vi "Sensor().vi"() -> (3 "Sensor.lvclass":refnum<class "Sensor.lvclass">)   [LabVIEW 2014, in "Sensors.lvlib" / "Sensor.lvclass"]
uses:
  Sensor.lvclass
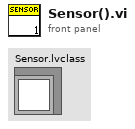
[diagram p1: front panel]
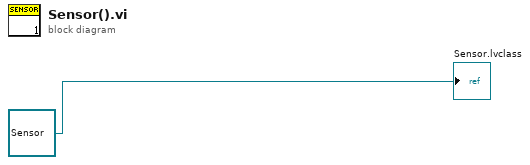
[diagram p0: block diagram]
diagram:
  "Sensor.lvclass" <- refnum<class "Sensor.lvclass"> refnum ("Sensor.lvclass")
